vi "Save VI at Path.vi"(5 "Save a Copy (F)":bool, 6 "Without Diagram (F)":bool, 7 "Override Existing? (T)":bool=TRUE, 8 "error in (no error)":errorcluster, 10 "Path":path, 11 "VI in":refnum<vi>) -> (0 "error out":errorcluster, 2 "Path to saved File":path, 3 "VI out":refnum<vi>)   [LabVIEW 2020, in "gRPC Scripting Tools.lvlib"]
uses:
  gRPC Scripting Tools.lvlib
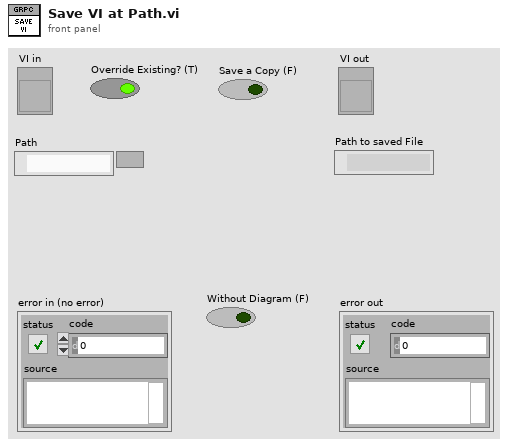
[diagram p1: front panel]
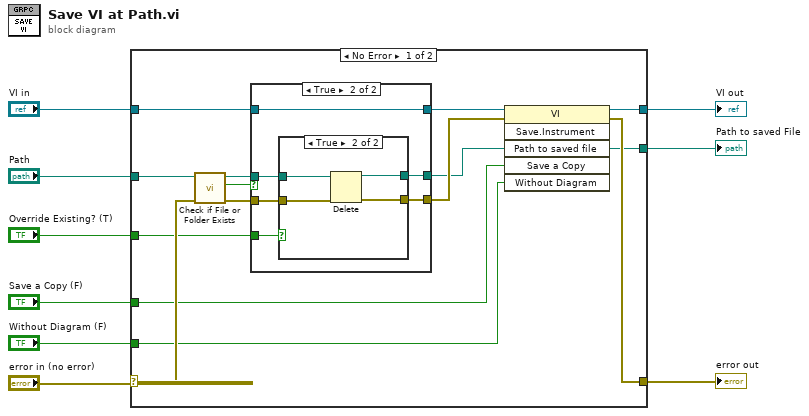
[diagram p0: block diagram]
diagram:
  n1 = case shown="No Error" "error in (no error)" {
    selector: "error in (no error)" -> [w21 w40]
    tunnel: "Path" -> [w22 w39]
    tunnel: "VI in" -> [w23 w41]
    tunnel: [w11 w40] -> w7
    tunnel: [w16 w41] -> w6
    tunnel: "Save a Copy (F)" -> [w13 _]
    tunnel: "Without Diagram (F)" -> [w12 _]
    tunnel: "Override Existing? (T)" -> [w15 _]
    tunnel: [w10 w39] -> w1
    frame No Error {
      n2 = call <vilib>:"Check if File or Folder Exists.vi"("error in (no error)"=w21, "path"=w22) -> ("error out"=w18:errorcluster, "file or folder exists?"=w19:bool, "dup path"=w20:path)  [unwired: 7 in]
      n3 = case shown="True" w19 {
        tunnel: w23 -> [w26 w32]
        tunnel: [w26 w32] -> w17
        tunnel: w20 -> [w24 w31]
        tunnel: w18 -> [w25 w30]
        tunnel: [w24 w29] -> w10
        tunnel: [w25 w28] -> w14
        tunnel: w15 -> [_ w27]
        frame False {
        }
        frame True {
          n4 = case shown="True" w27 {
            tunnel: w31 -> [w34 w38]
            tunnel: w30 -> [w33 w37]
            tunnel: [w34 w36] -> w29
            tunnel: [w33 w35] -> w28
            frame False {
            }
            frame True {
              n5 = Delete(path (use dialog)=w38, error in=w37) -> (deleted path=w36:path, error out=w35:errorcluster)  [unwired: 3 in, 1 out]
            }
          }
        }
      }
      n6 = invoke class="VI" method="Save.Instrument"(reference=w17, error in=w14, "Path to saved file"=w10, "Save a Copy"=w13, "Without Diagram"=w12) -> (reference out=w16:refnum<vi>, error out=w11:errorcluster)  [unwired: 1 in, 4 out]
    }
    frame Error {
    }
  }
  "error out" <- w7
  "VI out" <- w6
  "Path to saved File" <- w1
